vi "Create Temp.vi"(7 "Word In":bool[](array[boolean]), 8 "K":bool[](array[boolean]), 9 "F":bool[](array[boolean]), 10 "E":bool[](array[boolean]), 11 "A":bool[](array[boolean])) -> (3 "unsigned 32bit integer":u32 format="%b")   [LabVIEW 2013]
panel:
  in  "fixed-point type":fxp<+,9,9> format="%b"
  out "U8 Out":u8 format="%b"
  # "Test Case:\n\nA Irot 5:     00110001000100010000101101110100\nF:                10001011110000011101111100100001\nE:                11101001001001111110100110101011\nK:                11001010011000101100000111010110\nWord In:    10110111011010010100111100111110"
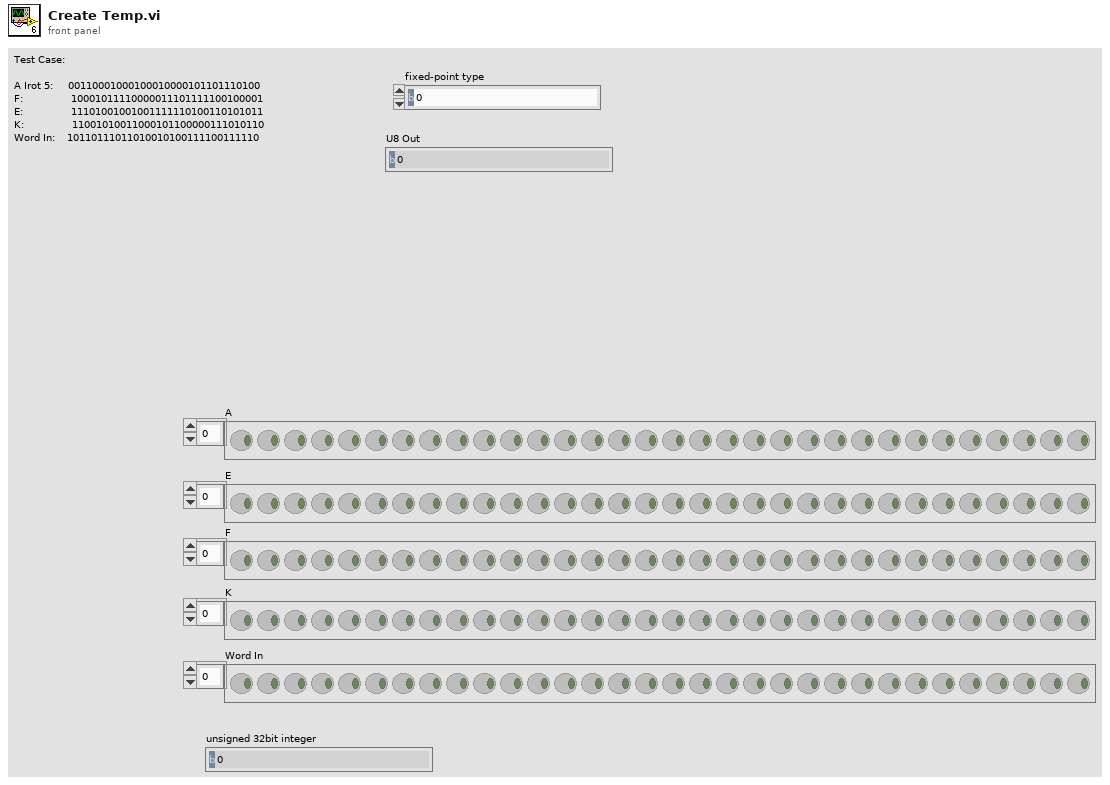
[diagram p1: front panel]
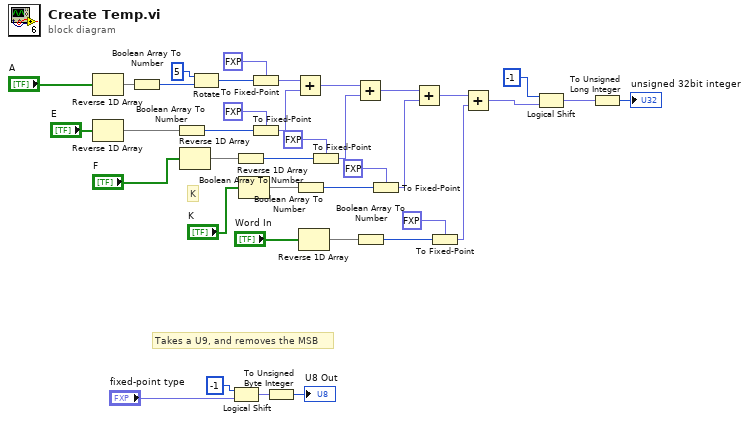
[diagram p0: block diagram]
diagram:
  # "Takes a U9, and removes the MSB"
  # "K"
  n1 = Reverse 1D Array(array="A") -> (reversed array=w10:bool[])
  n2 = Reverse 1D Array(array="E") -> (reversed array=w19:bool[])
  n3 = Boolean Array To Number(Boolean array=w10) -> (number=w11:u32)
  n4 = Boolean Array To Number(Boolean array=w19) -> (number=w16:u64)
  n5 = Reverse 1D Array(array="F") -> (reversed array=w20:bool[])
  n6 = Rotate(1:w11, 2:i16 5 ("y")) -> (0:w13:u32)
  n7 = Logical Shift(y=i16 -1, x="fixed-point type") -> (x << y=w6:fxp<+,9,9>)
  n8 = Boolean Array To Number(Boolean array=w20) -> (number=w22:u32)
  n9 = Reverse 1D Array(array="K") -> (reversed array=w29:bool[])
  n10 = To Fixed-Point(fixed-point type=fxp<+,36,36> 0.0, number=w13) -> (fixed-point=w24:fxp<+,36,36>)
  n11 = To Fixed-Point(fixed-point type=fxp<+,36,36> 0.0, number=w16) -> (fixed-point=w23:fxp<+,36,36>)
  n12 = To Unsigned Byte Integer(number=w6) -> (unsigned 8bit integer=→"U8 Out":u8)
  n13 = Add(x=w24, y=w23) -> (x+y=w25:fxp<+,37,37>)
  n14 = Boolean Array To Number(Boolean array=w29) -> (number=w30:u32)
  n15 = Reverse 1D Array(array="Word In") -> (reversed array=w36:bool[])
  n16 = To Fixed-Point(fixed-point type=fxp<+,36,36> 0.0, number=w22) -> (fixed-point=w26:fxp<+,36,36>)
  n17 = Add(x=w25, y=w26) -> (x+y=w27:fxp<+,38,38>)
  n18 = Boolean Array To Number(Boolean array=w36) -> (number=w35:u32)
  n19 = To Fixed-Point(fixed-point type=fxp<+,36,36> 0.0, number=w30) -> (fixed-point=w32:fxp<+,36,36>)
  n20 = Add(x=w27, y=w32) -> (x+y=w33:fxp<+,38,38>)
  n21 = To Fixed-Point(fixed-point type=fxp<+,36,36> 0.0, number=w35) -> (fixed-point=w38:fxp<+,36,36>)
  n22 = Add(x=w33, y=w38) -> (x+y=w2:fxp<+,39,39>)
  n23 = Logical Shift(y=i16 -1, x=w2) -> (x << y=w1:fxp<+,39,39>)
  n24 = To Unsigned Long Integer(number=w1) -> (unsigned 32bit integer=→"unsigned 32bit integer":u32)
